vi "AI_test1.vi"() -> ()   [LabVIEW 2016]
doc: "이 예제는 DAQmx 디바이스를 사용하여 버퍼있는 전류 측정값을 연속적으로 수집하는 방법을 보여줍니다.\n\n신호를 DAQ 디바이스에 연결하는 방법은 디바이스 문서를 참조하십시오."
uses:
  <vilib>/Utility/error.llb/DialogType.ctl
  <vilib>/DAQmx/read.llb/DAQmx Read (Analog 1D Wfm NChan NSamp).vi
  <vilib>/DAQmx/create/channels.llb/DAQmx Create Channel (AI-Voltage-Basic).vi
  <vilib>/DAQmx/configure/timing.llb/DAQmx Timing (Sample Clock).vi
  <vilib>/DAQmx/miscellaneous.llb/DAQmx Fill In Error Info.vi
  <resource>/objmgr/daqmx.rc
panel:
  out "Y":dbl[](array[numeric])
  out "dt":dbl
  out "t0":timestamp
  out "원소":waveform(dbl)
  out "data":waveform(dbl)[](array[waveform])
  in  "정지":bool
  out "웨이브폼 차트":waveform(dbl)[](graph)
  in  "루프 당 샘플":i32=1000
  in  "샘플 속도":dbl=1000.0
  in  "샘플 클럭 소스":tag="OnboardClock"
  in  "물리적 채널":tag="Dev1/ai0"
  out "실제 샘플 속도":dbl=1000.0 format="%0.2f"
  # "채널 셋팅"
  # "수집한 데이터"
  # "타이밍 셋팅"
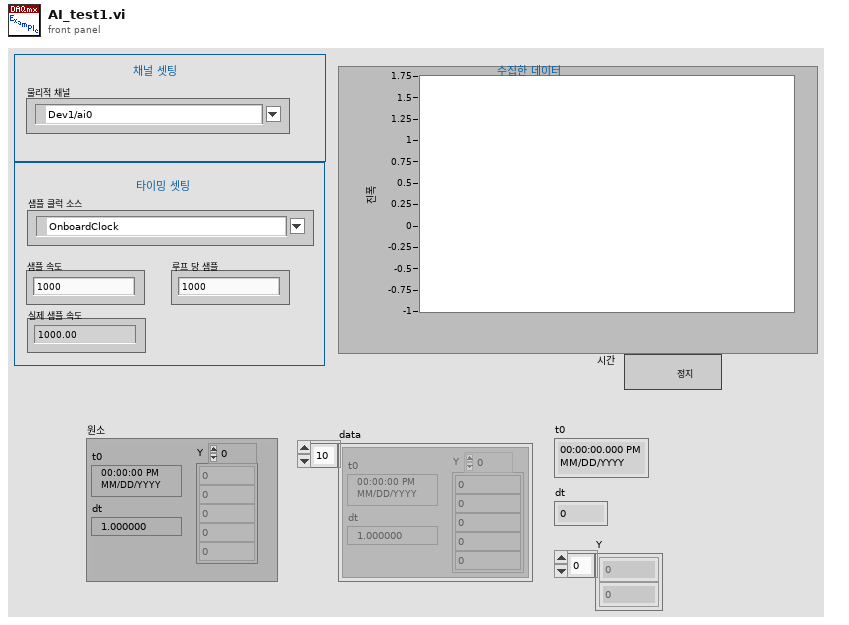
[diagram p1: front panel]
types:
  T1 = typedef "DialogType.ctl" = u16
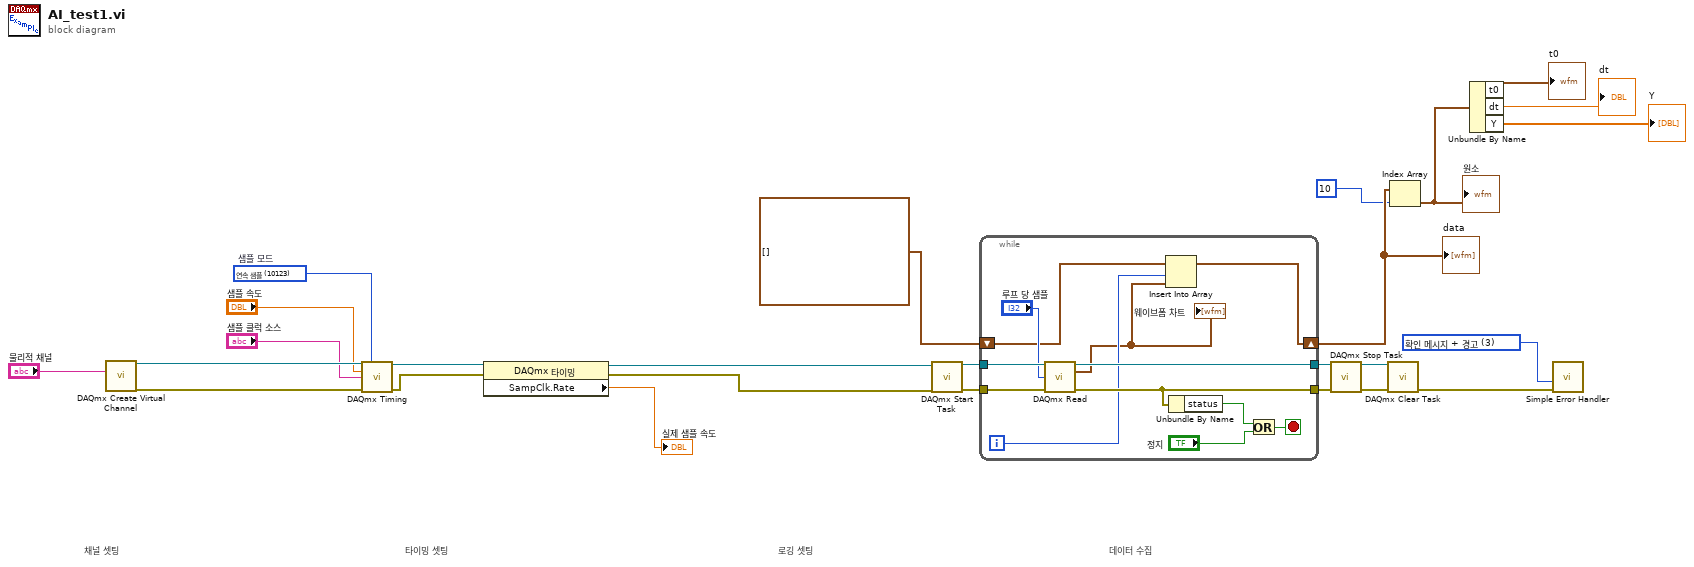
[diagram p0: block diagram]
diagram:
  w10 = T1 3 items=["대화 상자 없음", "확인 메시지", "메시지 지속 또는 정지", "확인 메시지 + 경고", "지속/정지 + 경고"] ("대화 상자 타입 (확인 메시지:1)")
  w24 = 10123 items=["유한 샘플"=10178, "연속 샘플"=10123, "하드웨어 타이밍에 의한 단일 포인트"=12522]  # 샘플 모드
  # "데이터 수집"
  # "타이밍 셋팅"
  # "채널 셋팅"
  # "로깅 셋팅"
  n1 = call-poly <vilib>:"DAQmx Create Virtual Channel.vi"("physical channels"="물리적 채널") -> ("task out"=w22:refnum<k21>, "error out"=w23:errorcluster)  [unwired: 13 in]
  n2 = call-poly <vilib>:"DAQmx Timing.vi"("task/channels in"=w22, "sample mode"=w24, "rate"="샘플 속도", "source"="샘플 클럭 소스", "error in"=w23) -> ("task out"=w26:refnum<k21>, "error out"=w25:errorcluster)  [unwired: 9 in]
  n3 = property class="DAQmx 타이밍"(reference=w26, error in=w25) -> (reference out=w8:refnum<k21>, error out=w9:errorcluster, "SampClk.Rate"=→"실제 샘플 속도":dbl)
  n4 = call <vilib>:"DAQmx Start Task.vi"("task/channels in"=w8, "error in"=w9) -> ("task out"=w21:refnum<k21>, "error out"=w20:errorcluster)  [unwired: 12 in]
  n5 = while {
    tunnel: w21 -> [w38]
    tunnel: w20 -> [w37]
    tunnel: [w34] -> w13
    tunnel: [w35] -> w14
    shift-right: [w27] -> w6
    shift-left: waveform(dbl)[] [] ("data") -> [w30]
    i -> [w29]
    stop <- w36 stop-if-true
    n6 = call-poly <vilib>:"DAQmx Read.vi"("task/channels in"=w38, "number of samples per channel"="루프 당 샘플", "error in"=w37) -> ("task out"=w35:refnum<k21>, "data"=w28:waveform(dbl)[], "error out"=w34:errorcluster)  [unwired: 10 in]
    "웨이브폼 차트" <- w28
    n7 = Insert Into Array(array=w30, index=w29, new element=w28) -> (w27:waveform(dbl)[])
    n8 = Unbundle By Name(w34) -> ("status"=w33:bool)
    n9 = Or(x=w33, y="정지") -> (x .or. y?=w36:bool)
  }
  "data" <- w6
  n10 = call <vilib>:"DAQmx Stop Task.vi"("task/channels in"=w14, "error in"=w13) -> ("task out"=w12:refnum<k21>, "error out"=w11:errorcluster)  [unwired: 12 in]
  n11 = call <vilib>:"DAQmx Clear Task.vi"("task in"=w12, "error in"=w11) -> ("error out"=w19:errorcluster)  [unwired: 13 in]
  n12 = Index Array(array=w6, index=10 ("인덱스")) -> (element=w4:waveform(dbl))
  "원소" <- w4
  n13 = Unbundle By Name(w4) -> ("t0"=→"t0":timestamp, "dt"=→"dt":dbl, "Y"=→"Y":dbl[])
  n14 = call <vilib>:"Simple Error Handler.vi"("type of dialog (OK msg:1)"=w10, "error in (no error)"=w19) -> ()  [unwired: 3 in, 5 out]
